vi "RunTimeMenu Custom Population.vi"(8 "error in (no error)":errorcluster, 10 "Menu Refnum":refnum<k9>, 11 "Node Ptr":u64 format="%.0x") -> (0 "error out":errorcluster)   [LabVIEW 2020, in "afdx_custom_device System Explorer.lvlib"]
uses:
  afdx_custom_device System Explorer.lvlib
  Includes/afdx_custom_device System Explorer.lvlibp/System Explorer/Implementation/System Explorer Dispatcher/System Explorer Dispatcher.lvclass
  C:/Users/Administrator/Downloads/vs-comms-bus-template/afdx_custom_device/Includes/afdx_custom_device System Explorer.lvlibp/System Explorer/Interfaces/System Explorer Dispatcher/System Explorer Dispatcher.lvclass
  Includes/afdx_custom_device System Explorer.lvlibp/System Explorer/Interfaces/System Explorer Dispatcher/System Explorer Dispatcher.lvclass
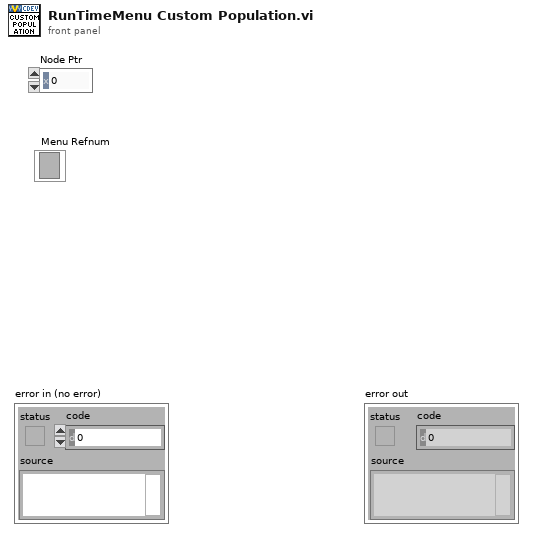
[diagram p1: front panel]
types:
  T1 = typedef "Custom Device API.lvlib/Custom Device Item Ref.ctl" = u64
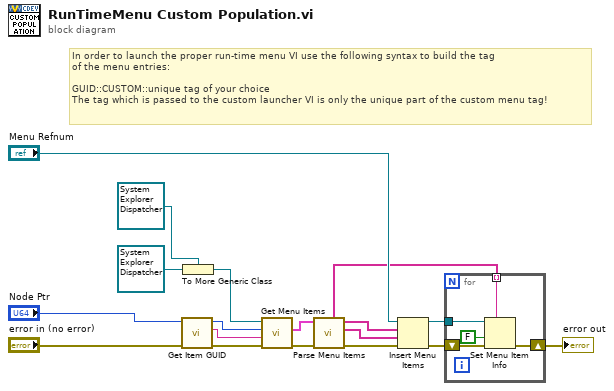
[diagram p0: block diagram]
diagram:
  # "In order to launch the proper run-time menu VI use the following syntax to build the tag\nof the menu entries:\n\nGUID::CUSTOM::unique tag of your choice\nThe tag which is passed to the custom launcher VI is only the unique part of the custom menu tag!"
  n1 = call "Get Item GUID.vi"("error in (no error)"="error in (no error)", "item in"="Node Ptr") -> ("error out"=w13:errorcluster, "guid"=w12:string, "item out"=w14:T1)  [unwired: 7 in]
  n2 = To More Generic Class(target class=refnum<class "System Explorer Dispatcher.lvclass"> refnum ("afdx_custom_device System Explorer.lvlibp:Interfaces.lvlib:System Explorer Dispatcher.lvclass"), reference=refnum<class "System Explorer Dispatcher.lvclass"> refnum ("afdx_custom_device System Explorer.lvlibp:Implementation.lvlib:System Explorer Dispatcher.lvclass")) -> (generic class reference=w17:refnum<class "System Explorer Dispatcher.lvclass">)
  n3 = call-dynamic "Get Menu Items.vi"("error in (no error)"=w13, "GUID"=w12, "Item Ref"=w14, "System Explorer Dispatcher in"=w17) -> ("error out"=w2:errorcluster, "Menu Items"=w11:cluster{"Name":string, "Enabled?":bool}[])  [unwired: 5 in, 1 out]
  n4 = call "Parse Menu Items.vi"("error in"=w2, "Menu Items"=w11) -> ("error out"=w1:errorcluster, "Item Tags"=w4:string[], "Item Names"=w5:string[], "Disabled Tags"=w3:string[])  [unwired: 6 in]
  n5 = Insert Menu Items(6:w1, 7:w4, 8:w5, 9:"Menu Refnum") -> (0:w7:errorcluster, 3:w8:refnum<k9>)  [unwired: 2 in, 1 out]
  n6 = for {
    tunnel: w8 -> [w23]
    shift-right: [w21] -> w6
    shift-left: w7 -> [w22]
    tunnel: w3 -> [w19] mode=indexing
    n7 = Set Menu Item Info(7:w19, 8:w22, 9:FALSE ("enabled"), 11:w23) -> (0:w21:errorcluster)  [unwired: 3 in, 1 out]
  }
  "error out" <- w6
